vi "Set Alarm Configuration.vi"(8 "error in":errorcluster, 10 "Alarm Configuration":T1 {"Alarm" items=["Alarm 1"=1, "Alarm 2"=2]}, 11 "CnPt in":refnum<class "CnPt.lvclass">) -> (0 "error out":errorcluster, 3 "CnPt out":refnum<class "CnPt.lvclass">)   [LabVIEW 2015, in "CnPt.lvclass"]
uses:
  CnPt.lvclass
  <vilib>/MSR Consulting, LLC/General Reuse/Session APIs/Serial/Serial Session.lvclass
  CnPt.lvclass/CnPt.ctl
  <vilib>/MSR Consulting, LLC/General Reuse/Session APIs/Serial/Public/Asynchronous Write.vi
  <vilib>/MSR Consulting, LLC/General Reuse/Session APIs/Serial/Public/Asynchronous Read.vi
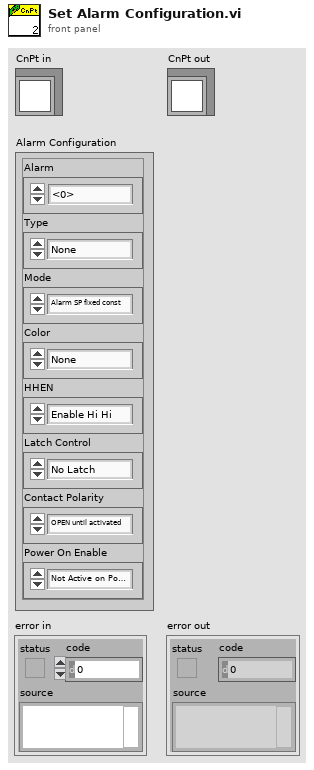
[diagram p1: front panel]
types:
  T1 = cluster{"Alarm":u16, "Type":enum16{"None", "PV > Alarm.H", "PV < Alarm.L", "PV > Alarm.H OR PV < Alarm.L", "PV < Alarm.H AND PV > Alarm.L"}, "Mode":enum16{"Alarm SP fixed const", "Alarm is offset from SP 1", "Alarm is offset from SP 2"}, "Color":enum16{"None", "GREEN", "RED", "AMBER"}, "HHEN":enum16{"Enable Hi Hi", "Disable Hi Hi"}, "Latch Control":enum16{"No Latch", "Clear by FP", "Clear by DI", "Clear by DI or FP"}, "Contact Polarity":enum16{"OPEN until activated", "CLOSED until activated"}, "Power On Enable":enum16{"Not Active on Power On", "Active On Power On"}}
  T2 = typedef "Serial Session.lvclass/Session Handle.ctl" = refnum<data-value>
  T3 = enum16{"None", "PV > Alarm.H", "PV < Alarm.L", "PV > Alarm.H OR PV < Alarm.L", "PV < Alarm.H AND PV > Alarm.L"}
  T4 = enum16{"Alarm SP fixed const", "Alarm is offset from SP 1", "Alarm is offset from SP 2"}
  T5 = enum16{"No Latch", "Clear by FP", "Clear by DI", "Clear by DI or FP"}
  T6 = enum16{"OPEN until activated", "CLOSED until activated"}
  T7 = enum16{"Not Active on Power On", "Active On Power On"}
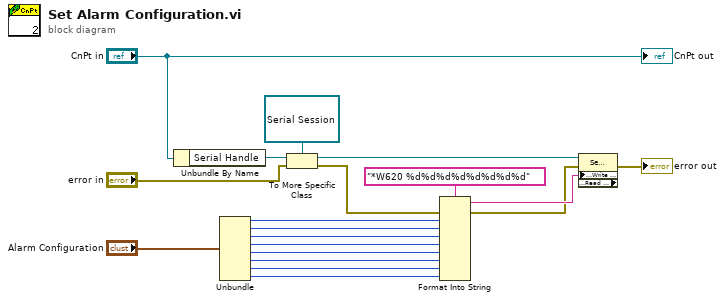
[diagram p0: block diagram]
diagram:
  n1 = Unbundle By Name("CnPt in") -> ("Serial Handle"=w19:T2)
  n2 = Unbundle("Alarm Configuration") -> ("Alarm"=w9:u16, "Type"=w8:T3, "Mode"=w7:T4, "Color"=w6:enum16{"None", "GREEN", "RED", "AMBER"}, "HHEN"=w5:enum16{"Enable Hi Hi", "Disable Hi Hi"}, "Latch Control"=w4:T5, "Contact Polarity"=w3:T6, "Power On Enable"=w1:T7)
  n3 = To More Specific Class(target class=refnum<data-value> refnum, reference=w19, error in="error in") -> (specific class reference=w17:refnum<data-value>, error out=w14:errorcluster)
  n4 = Format Into String(format string="*W620 %d%d%d%d%d%d%d%d", error in=w14, w9, w8, w7, w6, w5, w4, w3, w1) -> (resulting string=w15:string, error out=w13:errorcluster)  [unwired: 1 in]
  n5 = property class="Serial Session" props=["Public:Write - Asynchronous", "Public:Read - Asynchronous"](reference=w17, error in=w13, "Public:Write - Asynchronous"=w15) -> (error out=→"error out":errorcluster)  [unwired: 2 out]
  "CnPt out" <- "CnPt in"
